vi "Spark MAX Follow Custom.vi"(8 "error in (no error)":errorcluster, 10 "Follower Config":T6, 11 "MotorControlDeviceRef":T1) -> (0 "error out":errorcluster)   [LabVIEW 2023]
uses:
  c1a5a7da-df61-4eeb-b2f9-c2a549e58378.vi
  Typedef/Spark MAX Variant Data.ctl
  Typedef/SPARK CAN Arb ID.ctl
  Typedef/SPARK Model.ctl
  Typedef/Spark MAX Follower Config.ctl
  <vilib>/Rock Robotics/SystemInterfaces/DIO/FPGA_DIOPWMChannel.ctl
  <vilib>/Rock Robotics/WPI/PWM/WPI_PWMDeadband.ctl
  <vilib>/Rock Robotics/WPI/MotorControl/WPI_MotorControlType.ctl
  <vilib>/Rock Robotics/SystemInterfaces/DIO/FPGA_DIOChannel.ctl
  <vilib>/Rock Robotics/WPI/MotorControl/WPI_MotorControlDeviceRef.ctl
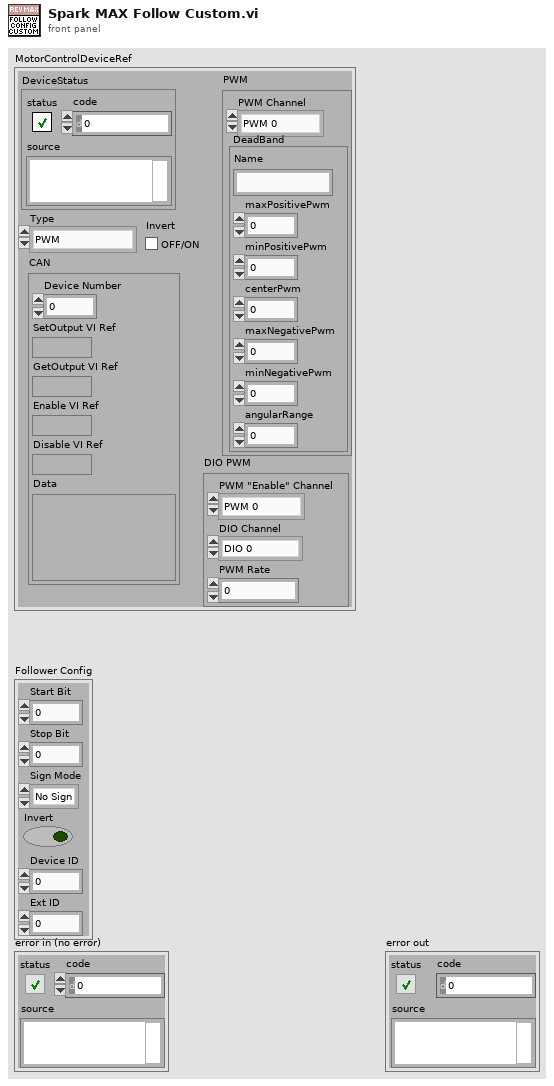
[diagram p1: front panel]
types:
  T1 = typedef "WPI_MotorControlDeviceRef.ctl" = cluster{"DeviceStatus":errorcluster, "Type":T2, "PWM":cluster{"PWM Channel":T3, "DeadBand":T4}, "CAN":cluster{"Device Number":u8, "SetOutput VI Ref":variant, "GetOutput VI Ref":variant, "Enable VI Ref":variant, "Disable VI Ref":variant, "Data":variant}, "Invert":bool, "DIO PWM":cluster{"PWM \"Enable\" Channel":T3, "DIOChannel":T5, "PWM Rate":dbl}}
  T2 = typedef "WPI_MotorControlType.ctl" = enum16{"PWM", "CAN", "DIO PWM"}
  T3 = typedef "FPGA_DIOPWMChannel.ctl" = enum8{"PWM 0", "PWM 1", "PWM 2", "PWM 3", "PWM 4", "PWM 5", "PWM 6", "PWM 7", "PWM 8", "PWM 9", "PWM MXP 0", "PWM MXP 1", "PWM MXP 2", "PWM MXP 3", "PWM MXP 4", "PWM MXP 5", "PWM MXP 6", "PWM MXP 7", "PWM MXP 8", "PWM MXP 9", "Invalid"}
  T4 = typedef "WPI_PWMDeadband.ctl" = cluster{"Name":string, "maxPositivePwm":i32, "minPositivePwm":i32, "centerPwm":i32, "maxNegativePwm":i32, "minNegativePwm":i32, "angularRange":u16}
  T5 = typedef "FPGA_DIOChannel.ctl" = enum8{"DIO 0", "DIO 1", "DIO 2", "DIO 3", "DIO 4", "DIO 5", "DIO 6", "DIO 7", "DIO 8", "DIO 9", "DIO MXP 0", "DIO MXP 1", "DIO MXP 2", "DIO MXP 3", "DIO MXP 4", "DIO MXP 5", "DIO MXP 6", "DIO MXP 7", "DIO MXP 8", "DIO MXP 9", "DIO MXP 10", "DIO MXP 11", "DIO MXP 12", "DIO MXP 13", "DIO MXP 14", "DIO MXP 15", "SPI Port CS1", "SPI Port CS2", "SPI Port CS3", "SPI Port MISO", "SPI Port MOSI", "Invalid"}
  T6 = typedef "Spark MAX Follower Config.ctl" = cluster{"Start Bit":u8, "Stop Bit":u8, "Sign Mode":enum16{"No Sign", "Twos Compliment", "Sign Magnitude"}, "Invert":bool, "Device ID":u8, "Ext ID":u32}
  T7 = typedef "SPARK CAN Arb ID.ctl" = u32
  T8 = typedef "Spark MAX Variant Data.ctl" = cluster{"Ext ID":u32, "CAN Timeout":u32, "Inverted No WPILib":bool, "Has Configured Limit Sw":bool, "Has Configured Alt Encoder":bool, "SPARK Model":T9, "CAN Max Retries":u32, "CAN Timeout (ms)":u32, "Status 0 Period (ms)":u32, "Status 1 Period (ms)":u32, "Status 2 Period (ms)":u32, "Status 3 Period (ms)":u32, "Status 4 Period (ms)":u32, "Status 5 Period (ms)":u32, "Status 6 Period (ms)":u32, "Status 7 Period (ms)":u32, "Status Frame Timeout (ms)":u32}
  T9 = typedef "SPARK Model.ctl" = enum16{"SPARK MAX", "SPARK Flex", "Unknown"}
  T10 = enum16{"No Sign", "Twos Compliment", "Sign Magnitude"}
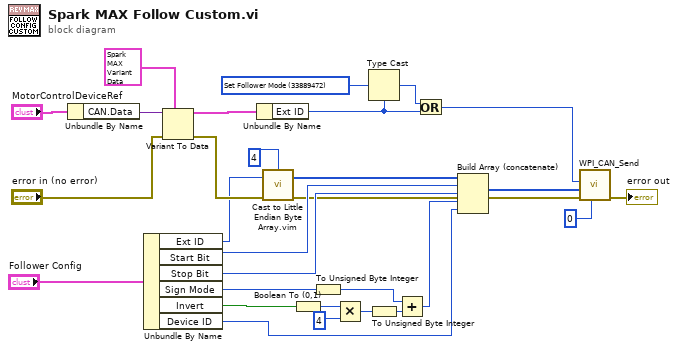
[diagram p0: block diagram]
diagram:
  w10 = T7 33889472 items=["Broadcast Disable"=0, "Broadcast System Halt"=64, "Broadcast System Reset"=128, "Broadcast Device Assign"=192, "Broadcast Heartbeat"=320, "Broadcast Firmware Version"=512, "Broadcast Enumerate"=576, "Broadcast System Resume"=640, "Duty Cycle Set"=33882240, "Speed Set"=33883264, "Position Set"=33885312, "Periodic Status 0"=33888256, "Periodic Status 1"=33888320, "User Status 0"=33888384, "User Status 1"=33888448, "User Status 2"=33888512, "User Status 3"=33888576, "DRV Status 0"=33888896, "DRV Status 1"=33888960, "Set Config Parameter"=33889280, "Get Config Parameter"=33889344, "Config Burn Flash"=33889408, "Set Follower Mode"=33889472, "Nack"=33890304, "Ack"=33890368, "Broadcast (not a command)"=33891328, "Heartbeat"=33891456, "Sync"=33891520, "IDQuery"=33891584, "IDAssign"=33891648] ("Parameter ID")
  n1 = Unbundle By Name("MotorControlDeviceRef") -> ("CAN.Data"=w6:variant)
  n2 = Unbundle By Name("Follower Config") -> ("Ext ID"=w1:u32, "Start Bit"=w18:u8, "Stop Bit"=w19:u8, "Sign Mode"=w24:T10, "Invert"=w20:bool, "Device ID"=w2:u8)
  n3 = Variant To Data(error in="error in (no error)", type=T8 {"Ext ID"=0, "CAN Timeout"=0, "Inverted No WPILib"=FALSE, "Has Configured Limit Sw"=FALSE, "Has Configured Alt Encoder"=FALSE, "SPARK Model"=enum."Unknown", "CAN Max Retries"=0, "CAN Timeout (ms)"=0, "Status 0 Period (ms)"=0, "Status 1 Period (ms)"=0, "Status 2 Period (ms)"=0, "Status 3 Period (ms)"=0, "Status 4 Period (ms)"=0, "Status 5 Period (ms)"=20, "Status 6 Period (ms)"=20, "Status 7 Period (ms)"=20, "Status Frame Timeout (ms)"=500} ("SPARK TNG Device Ref"), Variant=w6) -> (data=w5:T8, error out=w16:errorcluster)
  n4 = Unbundle By Name(w5) -> ("Ext ID"=w12:u32)
  n5 = call "Cast to Little Endian Byte Array.vim"("value"=w1, "bytes"=4) -> ("output array"=w13:u8[])  [unwired: 1 in]
  n6 = Boolean To (0,1)(Boolean=w20) -> (0, 1=w21:i16)
  n7 = To Unsigned Byte Integer(number=w24) -> (unsigned 8bit integer=w26:u8)
  n8 = Multiply(x=w21, y=i16 4) -> (x*y=w23:i16)
  n9 = Type Cast(type=w12, x=w10) -> (*(type *) &x=w11:u32)
  n10 = To Unsigned Byte Integer(number=w23) -> (unsigned 8bit integer=w25:u8)
  n11 = Add(x=w26, y=w25) -> (x+y=w27:u8)
  n12 = Or(x=w11, y=w12) -> (x .or. y?=w9:u32)
  n13 = Build Array (concatenate)(w13, w18, w19, w27, w2) -> (w14:u8[])
  n14 = call <vilib>:"WPI_CAN_Send.vi"("Period (ms)"=0, "error in (no error)"=w16, "Data"=w14, "Message ID"=w9) -> ("error out"=→"error out":errorcluster)  [unwired: 7 in]
